vi "FL Fuzzy Controller.vi"   [LabVIEW 2020, in "NI_Fuzzy_Logic_API.lvlib"]
doc: "Implements a fuzzy logic controller for the fuzzy system you specify."
uses:
  <vilib>/addons/Fuzzy Logic/NI_Fuzzy_Logic_API.lvlib
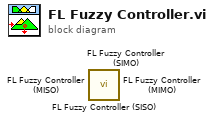
[diagram p0: block diagram]
diagram:
  n1 = call <vilib>:"FL Fuzzy Controller (SISO).vi"() -> ()  [unwired: 7 in, 5 out]
  n2 = call <vilib>:"FL Fuzzy Controller (SIMO).vi"() -> ()  [unwired: 7 in, 5 out]
  n3 = call <vilib>:"FL Fuzzy Controller (MISO).vi"() -> ()  [unwired: 7 in, 5 out]
  n4 = call <vilib>:"FL Fuzzy Controller (MIMO).vi"() -> ()  [unwired: 7 in, 5 out]
